vi "test - JSON Comparison - Cluster with Double and Array.vi"(8 "error in (no error)":errorcluster, 11 "TestCase in":refnum<class "Python Data Tools Tests.lvclass">) -> (0 "error out":errorcluster, 3 "TestCase out":refnum<class "Python Data Tools Tests.lvclass">)   [LabVIEW 2020, in "Python Data Tools Tests.lvclass"]
uses:
  Python Data Tools Tests.lvclass
  Python Data Tools Tests.lvclass/Python Data Tools Tests.ctl
  <vilib>/addons/_JKI Toolkits/VI Tester/TestCase.llb/TestCase.lvclass
  <userlib>/_OpenG.lib/time/time.llb/openg_time.lvlib
  C:/Program Files/National Instruments/LabVIEW 2020/vi.lib/addons/_JKI Toolkits/VI Tester/TestCase.llb/TestCase.lvclass
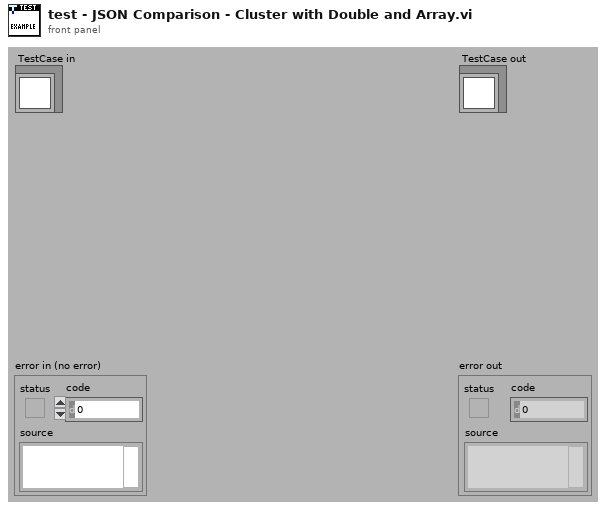
[diagram p1: front panel]
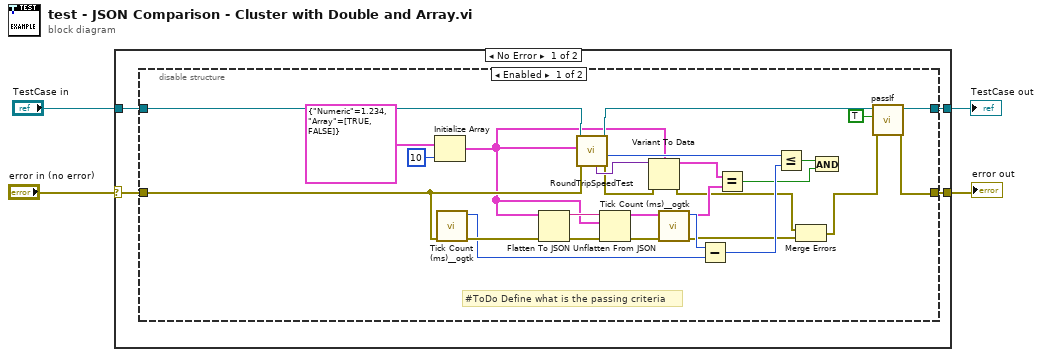
[diagram p0: block diagram]
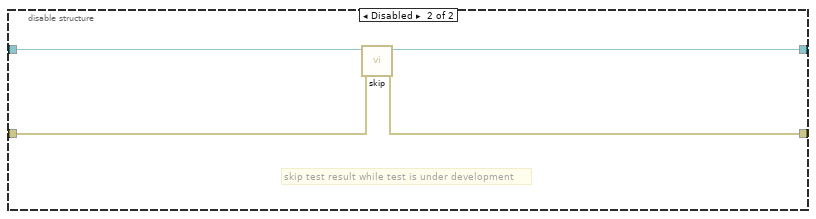
[diagram p2: hidden frame]
diagram:
  n1 = case shown="No Error" "error in (no error)" {
    selector: "error in (no error)" -> [w6 w40]
    tunnel: [w5 w40] -> w3
    tunnel: [w7 w39] -> w1
    tunnel: "TestCase in" -> [w8 w39]
    frame No Error {
      n2 = disable-structure shown="Enabled" {
        disable-tunnel: w8 -> [w34 w38]
        disable-tunnel: [w17 w35] -> w7
        disable-tunnel: w6 -> [w32 w37]
        disable-tunnel: [w15 w36] -> w5
        frame Enabled {
          # "#ToDo Define what is the passing criteria"
          n3 = Initialize Array(cluster{"Numeric":dbl, "Array":bool[]} {"Numeric"=1.234, "Array"=[TRUE, FALSE]}, 10 ("dimension size")) -> (w11:cluster{"Numeric":dbl, "Array":bool[]}[])
          n4 = call <userlib>:"Tick Count (ms)__ogtk.vi"("error in (no error)"=w32) -> ("error out"=w31:errorcluster, "millisecond timer value"=w27:u32)  [unwired: 9 in]
          n5 = Flatten To JSON(anything=w11, error in (no error)=w31) -> (JSON string=w33:string, 11:w29:errorcluster)  [unwired: 1 in]
          n6 = call "RoundTripSpeedTest.vi"("error in (no error)"=w32, "Variant"=w11, "TestCase in"=w34) -> ("error out"=w21:errorcluster, "Elapsed Time (ms)"=w26:u32, "TestCase out"=w18:refnum<class "Python Data Tools Tests.lvclass">, "data"=w24:variant)  [unwired: 4 in, 1 out]
          n7 = Unflatten From JSON(JSON string=w33, type and defaults=w11, error in (no error)=w29) -> (value=w22:cluster{"Numeric":dbl, "Array":bool[]}[], error out=w30:errorcluster)  [unwired: 4 in]
          n8 = Variant To Data(error in=w21, type=w11, Variant=w24) -> (data=w14:cluster{"Numeric":dbl, "Array":bool[]}[], error out=w19:errorcluster)
          n9 = call <userlib>:"Tick Count (ms)__ogtk.vi"("error in (no error)"=w30) -> ("error out"=w20:errorcluster, "millisecond timer value"=w28:u32)  [unwired: 9 in]
          n10 = Subtract(x=w28, y=w27) -> (x-y=w25:u32)
          n11 = Equal?(x=w14, y=w22) -> (x = y?=w13:bool)
          n12 = Less Or Equal?(x=w26, y=w25) -> (x <= y?=w23:bool)
          n13 = Merge Errors(w19, w20) -> (w16:errorcluster)
          n14 = And(x=w23, y=w13) -> ()  [unwired: 1 out]
          n15 = call-dynamic "passIf.vi"("error in (no error)"=w16, "pass"=TRUE, "TestCase in"=w18) -> ("error out"=w15:errorcluster, "TestCase out"=w17:refnum<class "Python Data Tools Tests.lvclass">)  [unwired: 7 in]
        }
        frame Disabled {
          # "skip test result while test is under development"
          n16 = call <vilib>:"skip.vi"("error in (no error)"=w37, "TestCase in"=w38) -> ("error out"=w36:errorcluster, "TestCase out"=w35:refnum<class "Python Data Tools Tests.lvclass">)  [unwired: 8 in]
        }
      }
    }
    frame Error {
    }
  }
  "error out" <- w3
  "TestCase out" <- w1
